vi "Hab Lifter Controller - PID.vi"(8 "error in":errorcluster) -> ()   [LabVIEW 2018]
doc: "This VI executes continuously carrying out the current operation and responding to updates or new operations. It will often contain the timing or control code that is difficult to place directly in TeleOp. This VI generally opens all sensors and motors and isolates the rest of the robot code from knowing how the operations are carried out."
uses:
  <vilib>/Rock Robotics/WPI/Framework/Completion Status.ctl
  Hab Lifter Setpoints.ctl
  Hab Lifter Operations.ctl
  <vilib>/Rock Robotics/WPI/ThirdParty/REV Robotics/SPARK MAX/Typedef/Spark MAX Control Type.ctl
panel:
  out "x-y":dbl
  out "Back Hab Velocity":dbl
  out "Front Hab Velocity":dbl
  in  "Interactive Values":T1
  out "Current\nCmd":string
  in  "Buttons":cluster{"Execute Cmd":bool, "Abort Cmd":bool}
  out "Command Timing":cluster{"Start Time (ms)":u32, "Iterations":i32}
  out "Status":T3
  # "Tip: It may be helpful to observe inputs and sensor values.\nYou may also want to display tuning or debugging controls."
  # "Click here to set max"
  # "Click here to set min"
  # "Interactive Command: You may fill in the settings for a command\nand schedule it with the Execute button. You can observe and abort\nany command while fine tuning the code for the controller."
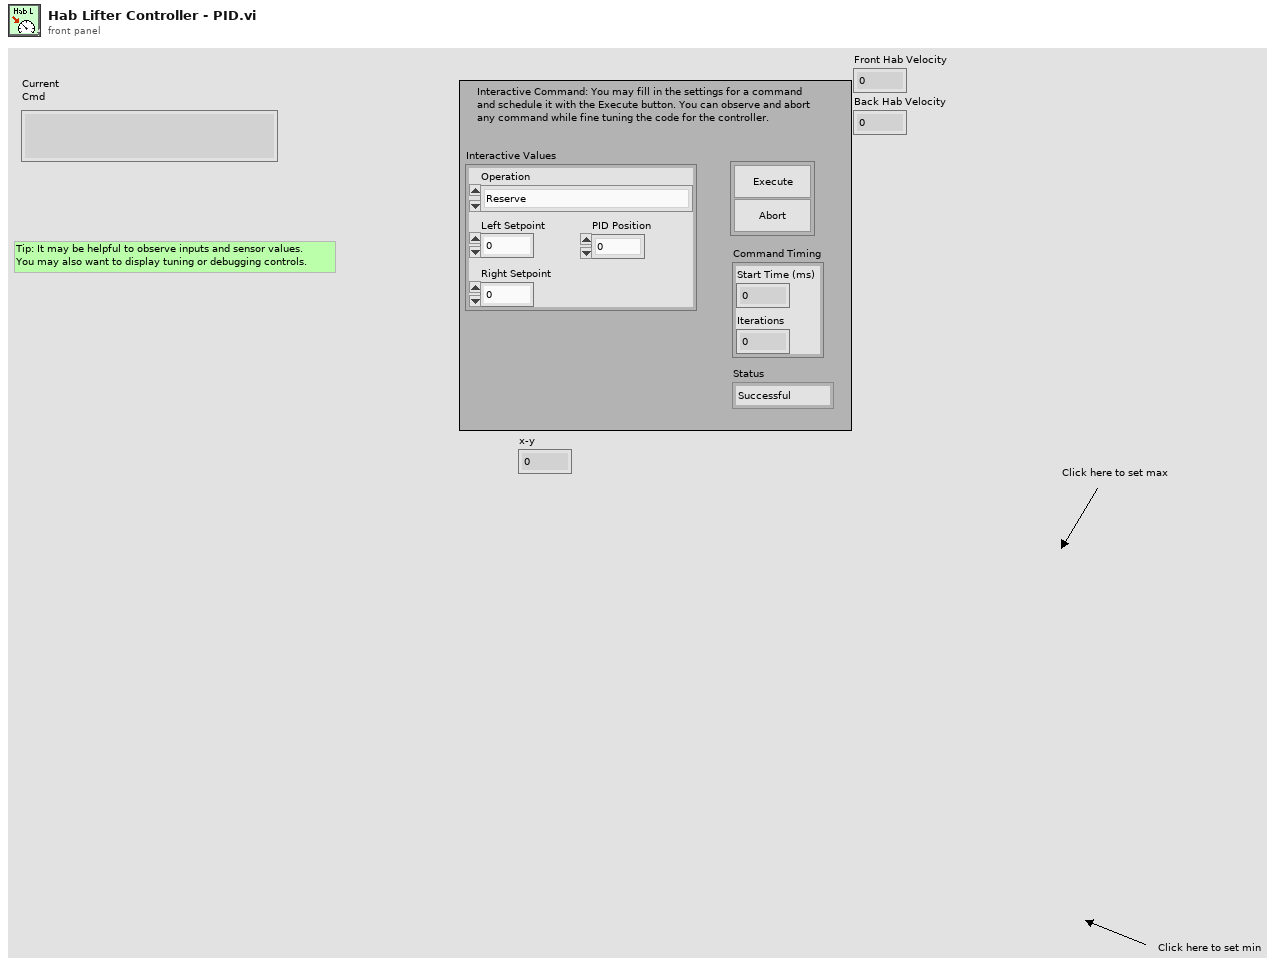
[diagram p1: front panel]
types:
  T1 = typedef "Hab Lifter Setpoints.ctl" = cluster{"Operation":T2, "Left Setpoint":dbl, "Right Setpoint":dbl, "PID Position":i16}
  T2 = typedef "Hab Lifter Operations.ctl" = enum16{"Reserve", "Read Current", "Immediate", "Immediate Simultaneous", "Yeah It's PID"}
  T3 = typedef "Completion Status.ctl" = enum16{"Successful", "Aborted", "Incomplete"}
  T4 = cluster{"P Gain":dbl, "I Gain":dbl, "D Gain":dbl, "F Gain":dbl, "I Zone":dbl, "Min Output":dbl, "Max Output":dbl}
  T5 = typedef "WPI_MotorControlDeviceRef.ctl" = cluster{"DeviceStatus":errorcluster, "Type":T6, "PWM":cluster{"PWM Channel":T7, "DeadBand":T8}, "CAN":cluster{"Device Number":u8, "SetOutput VI Ref":variant, "GetOutput VI Ref":variant, "Enable VI Ref":variant, "Disable VI Ref":variant, "Data":variant}, "Invert":bool, "DIO PWM":cluster{"PWM \"Enable\" Channel":T7, "DIOChannel":T9, "PWM Rate":dbl}}
  T6 = typedef "WPI_MotorControlType.ctl" = enum16{"PWM", "CAN", "DIO PWM"}
  T7 = typedef "FPGA_DIOPWMChannel.ctl" = enum8{"PWM 0", "PWM 1", "PWM 2", "PWM 3", "PWM 4", "PWM 5", "PWM 6", "PWM 7", "PWM 8", "PWM 9", "PWM MXP 0", "PWM MXP 1", "PWM MXP 2", "PWM MXP 3", "PWM MXP 4", "PWM MXP 5", "PWM MXP 6", "PWM MXP 7", "PWM MXP 8", "PWM MXP 9", "Invalid"}
  T8 = typedef "WPI_PWMDeadband.ctl" = cluster{"Name":string, "maxPositivePwm":i32, "minPositivePwm":i32, "centerPwm":i32, "maxNegativePwm":i32, "minNegativePwm":i32, "angularRange":u16}
  T9 = typedef "FPGA_DIOChannel.ctl" = enum8{"DIO 0", "DIO 1", "DIO 2", "DIO 3", "DIO 4", "DIO 5", "DIO 6", "DIO 7", "DIO 8", "DIO 9", "DIO MXP 0", "DIO MXP 1", "DIO MXP 2", "DIO MXP 3", "DIO MXP 4", "DIO MXP 5", "DIO MXP 6", "DIO MXP 7", "DIO MXP 8", "DIO MXP 9", "DIO MXP 10", "DIO MXP 11", "DIO MXP 12", "DIO MXP 13", "DIO MXP 14", "DIO MXP 15", "SPI Port CS1", "SPI Port CS2", "SPI Port CS3", "SPI Port MISO", "SPI Port MOSI", "Invalid"}
  T10 = typedef "Command Status Info.ctl" = cluster{"Name":string, "Status":T3, "notifier out":T11}
  T11 = typedef "Completion Notifier.ctl" = refnum<notifier>
  T12 = cluster{"Current Command":T1, "Command Timing":cluster{"Start Time (ms)":u32, "Iterations":i32}, "Command Arguments":cluster{"Command Info":T10, "Description":string, "Default Command":T1, "queue out":refnum<queue>, "Subsystem Name":string}}
  T13 = typedef "Spark MAX Control Type.ctl" = enum16{"Percent VBus", "Voltage", "Velocity", "Position", "Smart Motion", "Current"}
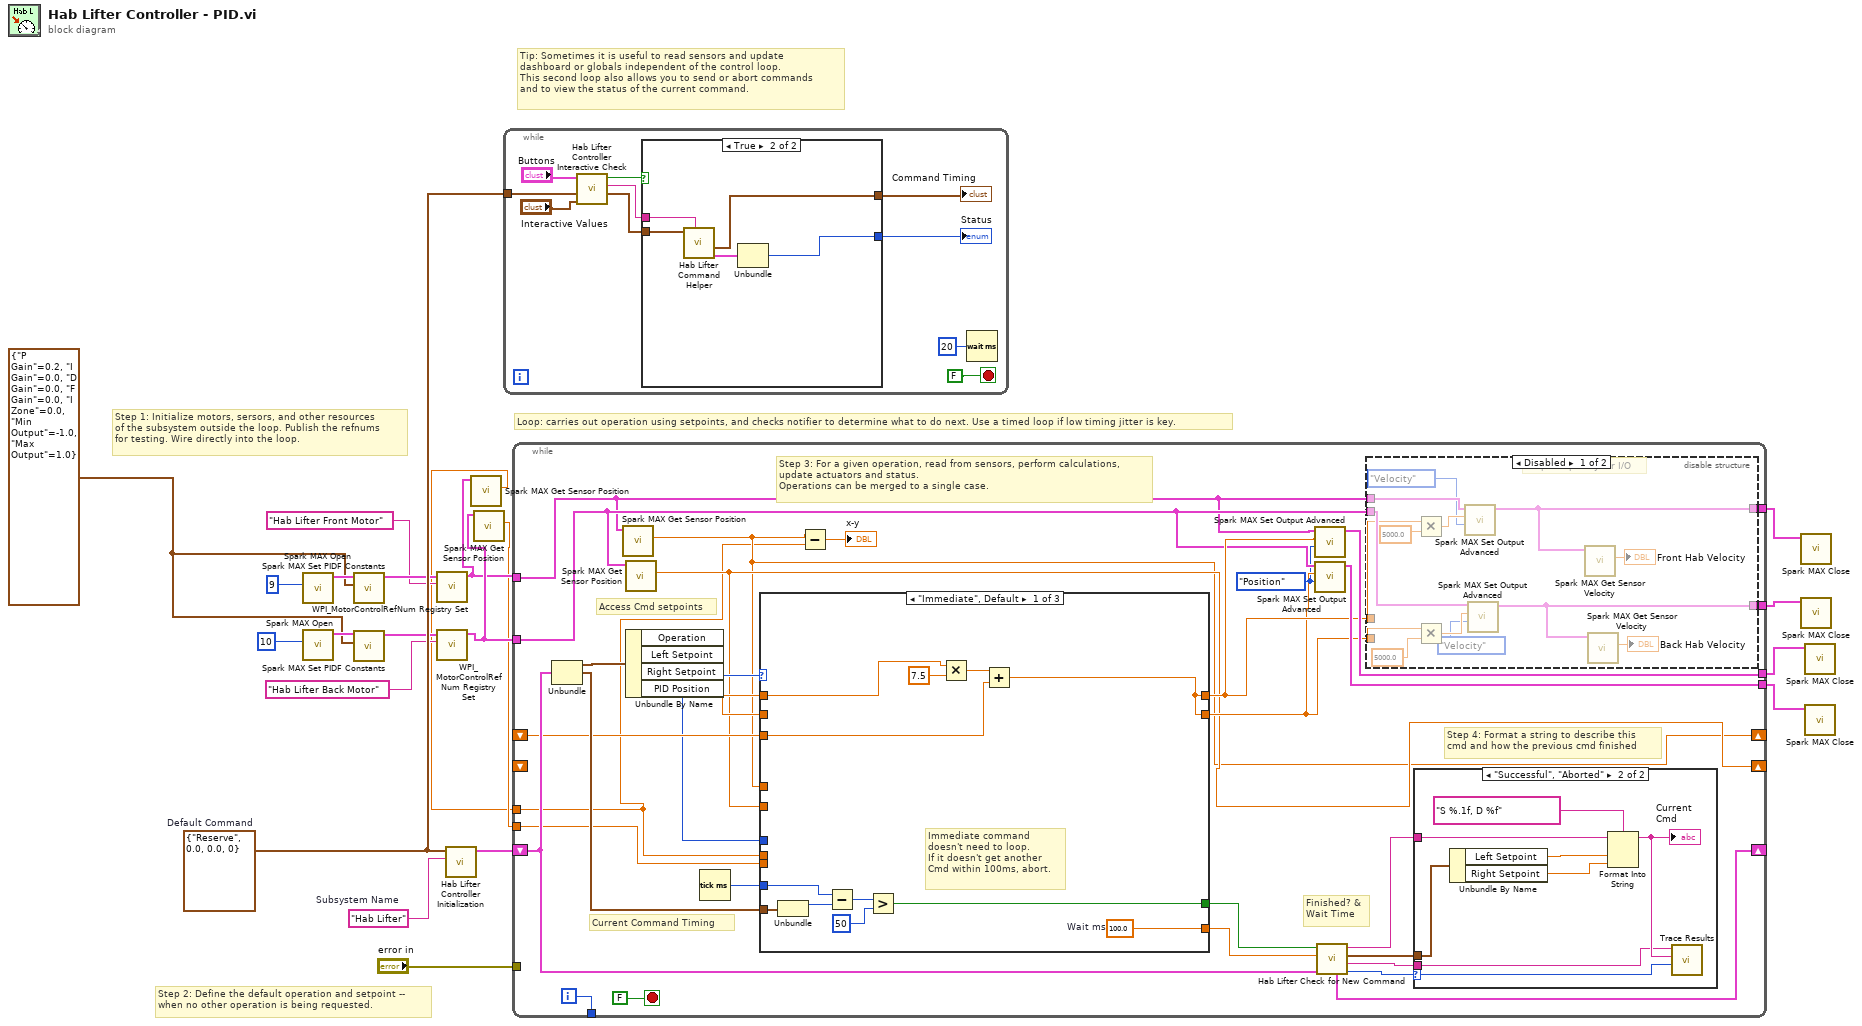
[diagram p0: block diagram]
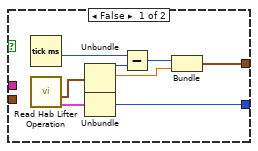
[diagram p2: hidden frame]
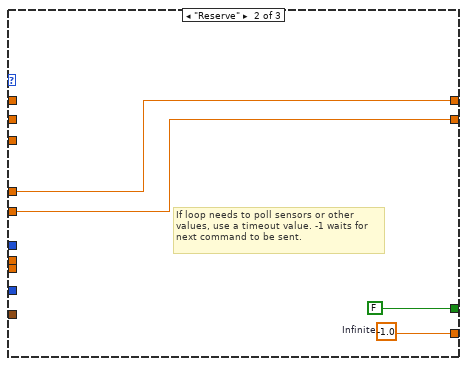
[diagram p5: hidden frame]
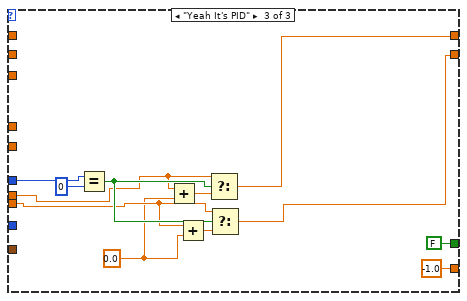
[diagram p6: hidden frame]
diagram:
  w13 = T4 {"P Gain"=0.2, "I Gain"=0.0, "D Gain"=0.0, "F Gain"=0.0, "I Zone"=0.0, "Min Output"=-1.0, "Max Output"=1.0} ("PID Constants")
  w18 = T1 {"Operation"=enum."Reserve", "Left Setpoint"=0.0, "Right Setpoint"=0.0, "PID Position"=0}  # Default Command
  w19 = "Hab Lifter"  # Subsystem Name
  # "Tip: Sometimes it is useful to read sensors and update\ndashboard or globals independent of the control loop.\nThis second loop also allows you to send or abort commands\nand to view the status of the current command."
  # "Step 2: Define the default operation and setpoint --\nwhen no other operation is being requested."
  # "Step 1: Initialize motors, sersors, and other resources\nof the subsystem outside the loop. Publish the refnums\nfor testing. Wire directly into the loop."
  # "Loop: carries out operation using setpoints, and checks notifier to determine what to do next. Use a timed loop if low timing jitter is key."
  n1 = call <vilib>:"Spark MAX Open.vi"("Device Number"=u8 9) -> ("MotorControlDeviceRef"=w17:T5)  [unwired: 9 in, 1 out]
  n2 = call <vilib>:"Spark MAX Open.vi"("Device Number"=u8 10) -> ("MotorControlDeviceRef"=w14:T5)  [unwired: 9 in, 1 out]
  n3 = call <vilib>:"Spark MAX Set PIDF Constants.vi"("PID Constants"=w13, "MotorControlDeviceRef"=w17) -> ("MotorControlDeviceRef"=w12:T5)  [unwired: 8 in, 1 out]
  n4 = call <vilib>:"Spark MAX Set PIDF Constants.vi"("PID Constants"=w13, "MotorControlDeviceRef"=w14) -> ("MotorControlDeviceRef"=w11:T5)  [unwired: 8 in, 1 out]
  n5 = call <vilib>:"WPI_MotorControlRefNum Registry Set.vi"("refnum name"="Hab Lifter Front Motor", "MotorControlDevRef"=w12) -> ("MotorControlDevRef"=w3:T5)  [unwired: 8 in, 1 out]
  n6 = call <vilib>:"WPI_MotorControlRefNum Registry Set.vi"("refnum name"="Hab Lifter Back Motor", "MotorControlDevRef"=w11) -> ("MotorControlDevRef"=w4:T5)  [unwired: 8 in, 1 out]
  n7 = call "Hab Lifter Controller Initialization.vi"("Subsystem Name"=w19, "Default Command"=w18) -> ("Current Command"=w20:T12)  [unwired: 9 in]
  n8 = call <vilib>:"Spark MAX Get Sensor Position.vi"("MotorControlDevRef in"=w3) -> ("Sensor Position"=w1:dbl)  [unwired: 7 in, 3 out]
  n9 = call <vilib>:"Spark MAX Get Sensor Position.vi"("MotorControlDevRef in"=w4) -> ("Sensor Position"=w2:dbl)  [unwired: 7 in, 3 out]
  n10 = while {
    tunnel: w18 -> [w28]
    stop <- FALSE stop-if-true
    n11 = call "Hab Lifter Controller Interactive Check.vi"("Interactive Command in"="Interactive Values", "Default Command"=w28, "Buttons"="Buttons") -> ("Interactive Command out"=w25:T1, "Trace String"=w26:string, "Schedule"=w27:bool)  [unwired: 6 in]
    n12 = case shown="True" w27 {
      tunnel: [w39 w44] -> w24
      tunnel: w25 -> [_ w42]
      tunnel: [w35 w40] -> w23
      tunnel: w26 -> [_ w43]
      frame False {
        n13 = Tick Count (ms)() -> (millisecond timer value=w34:u32)
        n14 = call "Read Hab Lifter Operation.vi"() -> ("Command Info"=w32:T10, "SubSystem Data"=w33:T1)  [unwired: 9 in, 1 out]
        n15 = Unbundle(w33) -> ("Operation"=w38:T2, "Left Setpoint"=w36:dbl)  [unwired: 2 out]
        n16 = Unbundle(w32) -> ("Status"=w39:T3)  [unwired: 2 out]
        n17 = Subtract(x=w34, y=w38) -> (x-y=w37:u32)
        n18 = Bundle(w37, "Left Setpoint"=w36) -> (w35:cluster{u32, "Left Setpoint":dbl})  [unwired: 1 in]
      }
      frame True {
        n19 = call "Hab Lifter Command Helper.vi"("Description"=w43, "SubSystem Data"=w42) -> ("Command Info Out"=w41:T10, "Command Timing"=w40:cluster{"Start Time (ms)":u32, "Iterations":i32})  [unwired: 7 in, 1 out]
        n20 = Unbundle(w41) -> ("Status"=w44:T3)  [unwired: 2 out]
      }
    }
    "Status" <- w24
    "Command Timing" <- w23
    n21 = Wait (ms)(milliseconds to wait=u32 20) -> ()  [unwired: 1 out]
  }
  n22 = while {
    shift-right: [w68] -> _
    shift-left: w20 -> [w61]
    tunnel: [w75] -> _
    tunnel: "error in" -> [_]
    tunnel: w3 -> [w53]
    tunnel: w4 -> [w54]
    tunnel: [w60] -> w8
    tunnel: [w59] -> w7
    tunnel: [w57] -> w6
    tunnel: [w58] -> w5
    shift-right: [w47] -> _
    shift-left: _ -> [w51]
    shift-right: [w50] -> _
    shift-left: _ -> [_]
    tunnel: w2 -> [w48]
    tunnel: w1 -> [w46]
    i -> [w75]
    stop <- FALSE stop-if-true
    w52 = Spark_MAX_Control_Type."Position" ("Control Mode")
    # "Step 4: Format a string to describe this\ncmd and how the previous cmd finished"
    # "Current Command Timing"
    # "Access Cmd setpoints"
    # "Finished? &\nWait Time"
    # "Step 3: For a given operation, read from sensors, perform calculations,\nupdate actuators and status.\nOperations can be merged to a single case."
    n23 = Unbundle(w61) -> ("Current Command"=w74:T1, "Command Timing"=w70:cluster{"Start Time (ms)":u32, "Iterations":i32})  [unwired: 1 out]
    n24 = call <vilib>:"Spark MAX Get Sensor Position.vi"("MotorControlDevRef in"=w53) -> ("Sensor Position"=w47:dbl)  [unwired: 7 in, 3 out]
    n25 = call <vilib>:"Spark MAX Get Sensor Position.vi"("MotorControlDevRef in"=w54) -> ("Sensor Position"=w50:dbl)  [unwired: 7 in, 3 out]
    n26 = Unbundle By Name(w74) -> ("Operation"=w73:T2, "Left Setpoint"=w72:dbl, "Right Setpoint"=w69:dbl, "PID Position"=w49:i16)
    n27 = Tick Count (ms)() -> (millisecond timer value=w71:u32)
    n28 = case shown="\"Immediate\", Default" w73 {
      tunnel: [w110 w114 -1.0 ("Infinite")] -> w66
      tunnel: [w104 FALSE ("ignore previous (F)") FALSE ("ignore previous (F)")] -> w67
      tunnel: w70 -> [w106 _ _]
      tunnel: w72 -> [w100 _ _]
      tunnel: w71 -> [w105 _ _]
      tunnel: w69 -> [_ _ _]
      tunnel: [w102 w111 w122] -> w55
      tunnel: [w102 w112 w121] -> w56
      tunnel: w47 -> [_ w112 _]
      tunnel: w50 -> [_ w111 _]
      tunnel: w51 -> [w103 _ _]
      tunnel: w49 -> [_ _ w124]
      tunnel: w46 -> [_ _ w117]
      tunnel: w48 -> [_ _ w116]
      frame "Immediate", Default {
        w110 = 100.0  # Wait ms
        # "Immediate command\ndoesn't need to loop.\nIf it doesn't get another\nCmd within 100ms, abort."
        n29 = Unbundle(w106) -> ("Start Time (ms)"=w109:u32)  [unwired: 1 out]
        n30 = Subtract(x=w105, y=w109) -> (x-y=w108:u32)
        n31 = Greater?(x=w108, y=u8 50 ("Left Motor")) -> (0:w104:bool)
        n32 = Multiply(x=w100, y=7.5) -> (x*y=w99:dbl)
        n33 = Add(x=w99, y=w103) -> (x+y=w102:dbl)
      }
      frame "Reserve" {
        w114 = -1.0  # Infinite
        # "If loop needs to poll sensors or other\nvalues, use a timeout value. -1 waits for\nnext command to be sent."
      }
      frame "Yeah It's PID" {
        w115 = 0.0
        n34 = Equal?(x=w124, y=i16 0) -> (x = y?=w120:bool)
        n35 = Add(x=w117, y=w115) -> (x+y=w118:dbl)
        n36 = Add(x=w116, y=w115) -> (x+y=w119:dbl)
        n37 = Select(t=w117, s=w120, f=w118) -> (s? t:f=w121:dbl)
        n38 = Select(t=w116, s=w120, f=w119) -> (s? t:f=w122:dbl)
      }
    }
    n39 = Subtract(x=w47, y=w46) -> (x-y=→"x-y":dbl)
    n40 = call <vilib>:"Spark MAX Set Output Advanced.vi"("Control Mode"=w52, "Setpoint"=w56, "MotorControlDevRef"=w53) -> ("MotorControlDevRef"=w57:T5)  [unwired: 7 in, 1 out]
    n41 = call <vilib>:"Spark MAX Set Output Advanced.vi"("Control Mode"=w52, "Setpoint"=w55, "MotorControlDevRef"=w54) -> ("MotorControlDevRef"=w58:T5)  [unwired: 7 in, 1 out]
    n42 = call "Hab Lifter Check for New Command.vi"("Current Command"=w61, "Wait time (ms)"=w66, "Finished?"=w67) -> ("Completion"=w62:T3, "Subsystem Name"=w63:string, "Current Command"=w64:T1, "Initial Trace String"=w65:string, "NextCommand"=w68:T12)  [unwired: 4 in]
    n43 = disable-structure shown="Disabled" {
      disable-tunnel: w53 -> [w90 _]
      disable-tunnel: w54 -> [w89 _]
      disable-tunnel: w56 -> [w88 _]
      disable-tunnel: w55 -> [w87 _]
      disable-tunnel: [w80 _] -> w60
      disable-tunnel: [w79 _] -> w59
      frame Disabled {
        # "Step 5: Upate your I/O"
        n44 = Multiply(x=w88, y=5000.0) -> (x*y=w85:dbl)
        n45 = Multiply(x=w87, y=5000.0) -> (x*y=w82:dbl)
        n46 = call <vilib>:"Spark MAX Set Output Advanced.vi"("Control Mode"=Spark_MAX_Control_Type."Velocity", "Setpoint"=w85, "MotorControlDevRef"=w90) -> ("MotorControlDevRef"=w80:T5)  [unwired: 7 in, 1 out]
        n47 = call <vilib>:"Spark MAX Set Output Advanced.vi"("Control Mode"=Spark_MAX_Control_Type."Velocity", "Setpoint"=w82, "MotorControlDevRef"=w89) -> ("MotorControlDevRef"=w79:T5)  [unwired: 7 in, 1 out]
        n48 = call <vilib>:"Spark MAX Get Sensor Velocity.vi"("MotorControlDevRef in"=w80) -> ("Sensor Velocity"=→"Front Hab Velocity":dbl)  [unwired: 7 in, 3 out]
        n49 = call <vilib>:"Spark MAX Get Sensor Velocity.vi"("MotorControlDevRef in"=w79) -> ("Sensor Velocity"=→"Back Hab Velocity":dbl)  [unwired: 7 in, 3 out]
      }
      frame Enabled {
      }
    }
    n50 = case shown="\"Successful\", \"Aborted\"" w62 {
      selector: w62 -> [_ w98]
      tunnel: w65 -> [_ w94]
      tunnel: w64 -> [_ w95]
      tunnel: w63 -> [_ w91]
      frame "Incomplete", Default {
        # "Continuing current command"
      }
      frame "Successful", "Aborted" {
        # "Report and setup for next command"
        n51 = Unbundle By Name(w95) -> ("Left Setpoint"=w97:dbl, "Right Setpoint"=w92:dbl)
        n52 = Format Into String(format string="S %.1f, D %f", initial string=w94, w97, w92) -> (resulting string=w93:string)  [unwired: 1 in, 1 out]
        "Current\nCmd" <- w93
        n53 = call <vilib>:"Trace Results.vi"("Status of previous command"=w98, "Description"=w93, "Subsystem"=w91) -> ()  [unwired: 9 in]
      }
    }
  }
  n54 = call <vilib>:"Spark MAX Close.vi"("MotorControlDeviceRef"=w8) -> ()  [unwired: 10 in, 1 out]
  n55 = call <vilib>:"Spark MAX Close.vi"("MotorControlDeviceRef"=w7) -> ()  [unwired: 10 in, 1 out]
  n56 = call <vilib>:"Spark MAX Close.vi"("MotorControlDeviceRef"=w6) -> ()  [unwired: 10 in, 1 out]
  n57 = call <vilib>:"Spark MAX Close.vi"("MotorControlDeviceRef"=w5) -> ()  [unwired: 10 in, 1 out]
